vi "DMM Panel.vi"(8 "error in (no error)":errorcluster, 9 "DMM Configuration (\"\")":string, 10 "DMM Stimulus":T3, 11 "DMM Command":T1=enum."MEASURE") -> (0 "error out":errorcluster, 1 "DMM Flat Output":string, 2 "DMM Measurement":T2 caption="This reading is allways in the base units\ni.e. V, A, Ohms, Hz, Sec, etc." format="%#_10f")   [LabVIEW 2011]
uses:
  DMM Measurement.ctl
  tests/DC Attenuation/TypeDefs/DCA Stimulus Parameters.ctl
  DMM Command.ctl
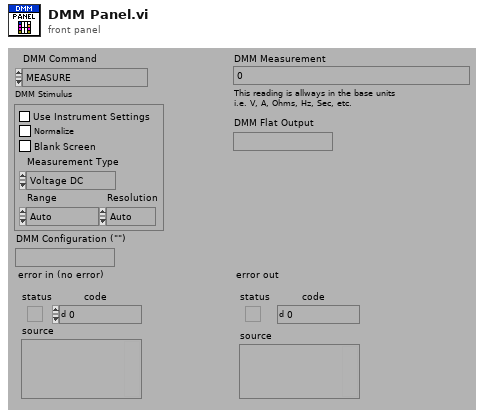
[diagram p1: front panel]
types:
  T1 = typedef "DMM Command.ctl" = enum16{"LOAD", "INITIALIZE", "PRESET", "GET STIMULUS", "SET STIMULUS", "MEASURE", "RELEASE", "UNLOAD", "GET CALIBRATION", "CALIBRATE"}
  T2 = typedef "DMM Measurement.ctl" = dbl
  T3 = typedef "DCA Stimulus Parameters.ctl" = cluster{"Use Instrument":bool, "Normalize":bool, "Blank Screen":bool, "Measurement Type":enum16{"Voltage DC", "Voltage DC Ratio", "Voltage AC", "Current DC", "Current AC", "Resistance", "Fresistance", "Frequency", "Period", "Continuity", "Diode"}, "Range":enum16{"Auto", "Minimum", "Maximum", "100", "1,000", "10,000", "100,000", "1,000,000", "10,000,000", "100,000,000"}, "Resolution":enum16{"Auto", "4 1/2", "5 1/2", "6 1/2"}}
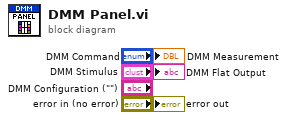
[diagram p0: block diagram]
diagram:
